vi "Read status.vi"(8 "error in (no error)":errorcluster, 11 "TCSCommand in":refnum<class "TCSCommand.lvclass">) -> (0 "error out":errorcluster, 2 "status":bool, 3 "TCSCommand out":refnum<class "TCSCommand.lvclass">)   [LabVIEW 2022 SP3, in "TCSDataDefinitions.lvlib" / "TCSCommand.lvlib" / "TCSCommand.lvclass"]
uses:
  TCSCommand.lvclass
  TCSCommand.lvclass/TCSCommand.ctl
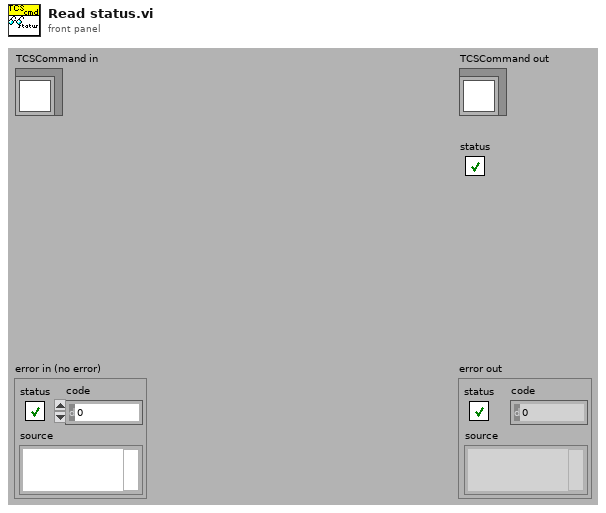
[diagram p1: front panel]
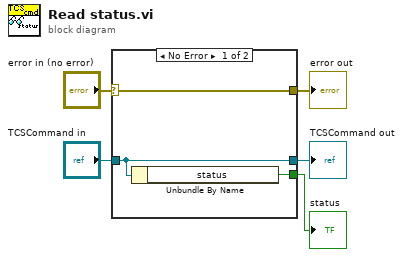
[diagram p0: block diagram]
diagram:
  n1 = case shown="No Error" "error in (no error)" {
    selector: "error in (no error)" -> [w8 w9]
    tunnel: [w8 w9] -> w4
    tunnel: [w7 w10] -> w2
    tunnel: "TCSCommand in" -> [w7 w10]
    tunnel: [w6 _] -> w1
    frame No Error {
      n2 = Unbundle By Name(w7) -> ("status"=w6:bool)
    }
    frame Error {
    }
  }
  "error out" <- w4
  "TCSCommand out" <- w2
  "status" <- w1
